vi "BattreyFGV.vi"(7 "Enum":enum16{"初始化", "讀取", "寫入", "閒置"}(ring), 10 "File Path":path=path "D:/battery/positive.txt", 11 "電池正負極陣列(輸入)":bool[](array[boolean])=[TRUE, TRUE, TRUE, TRUE, TRUE, TRUE, TRUE, TRUE, TRUE, TRUE, TRUE, TRUE, TRUE, TRUE, TRUE, TRUE, TRUE, TRUE, TRUE, TRUE, TRUE, TRUE, TRUE, TRUE, TRUE, TRUE, TRUE, TRUE, TRUE, TRUE, TRUE, TRUE, TRUE, TRUE, TRUE, TRUE, TRUE, TRUE, TRUE, TRUE]) -> (3 "電池正負極陣列(輸出)":bool[](array[boolean])=[TRUE, FALSE, TRUE, FALSE, TRUE, FALSE, TRUE, FALSE, TRUE, FALSE, TRUE, TRUE, FALSE, TRUE, FALSE, TRUE, FALSE, FALSE, TRUE, FALSE, TRUE, FALSE, TRUE, TRUE, FALSE, TRUE, FALSE, TRUE, FALSE, FALSE, TRUE, FALSE, TRUE, FALSE, TRUE, FALSE, TRUE, FALSE, TRUE, FALSE])   [LabVIEW 2015]
panel:
  in  "error In":errorcluster
  out "error out":errorcluster
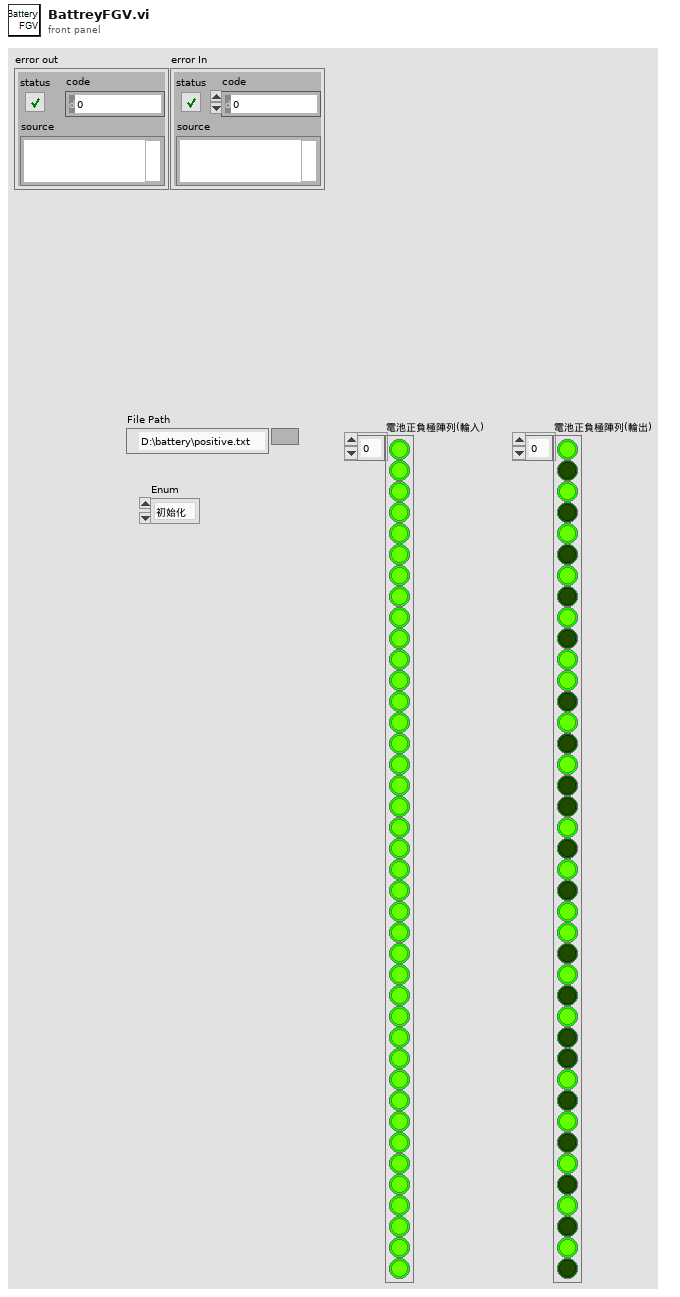
[diagram p1: front panel]
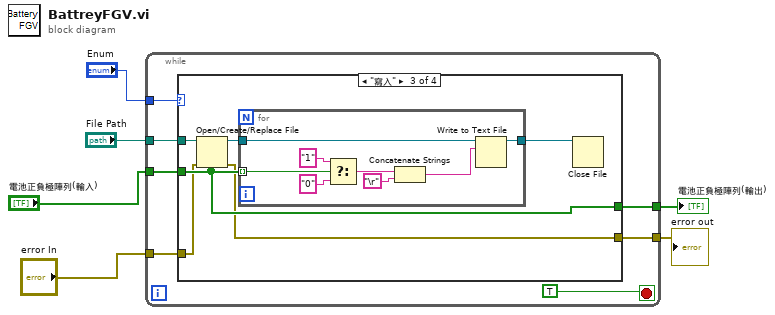
[diagram p0: block diagram]
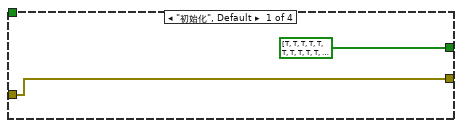
[diagram p2: hidden frame]
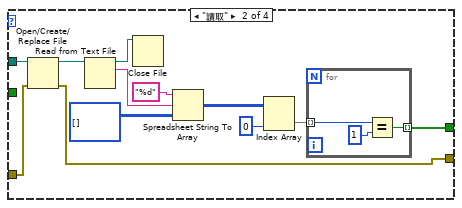
[diagram p3: hidden frame]
diagram:
  n1 = while {
    tunnel: "Enum" -> [w13]
    tunnel: "File Path" -> [w12]
    tunnel: [w11] -> w4
    tunnel: "電池正負極陣列(輸入)" -> [w10]
    tunnel: [w8] -> w2
    tunnel: "error In" -> [w7]
    stop <- TRUE stop-if-true
    n2 = case shown="\"寫入\"" w13 {
      tunnel: w12 -> [_ w19 w34 _]
      tunnel: [bool[] [TRUE, TRUE, TRUE, TRUE, TRUE, TRUE, TRUE, TRUE, TRUE, TRUE, TRUE, TRUE, TRUE, TRUE, TRUE, TRUE, TRUE, TRUE, TRUE, TRUE, TRUE, TRUE, TRUE, TRUE, TRUE, TRUE, TRUE, TRUE, TRUE, TRUE, TRUE, TRUE, TRUE, TRUE, TRUE, TRUE, TRUE, TRUE, TRUE, TRUE] ("電池正負極陣列(輸入)") w18 w33 w46] -> w11
      tunnel: w10 -> [_ _ w33 w46]
      tunnel: [w14 w17 w31 w45] -> w8
      tunnel: w7 -> [w14 w16 w32 w45]
      frame "初始化", Default {
      }
      frame "讀取" {
        n3 = Open/Create/Replace File(file path (use dialog)=w19, error in=w16) -> (refnum out=w25:refnum<file>, error out=w17:errorcluster)  [unwired: 4 in, 1 out]
        n4 = Read from Text File(file (use dialog)=w25) -> (refnum out=w22:refnum<file>, text=w27:string)  [unwired: 3 in, 2 out]
        n5 = Close File(refnum=w22) -> ()  [unwired: 1 in, 2 out]
        n6 = Spreadsheet String To Array(format string="%d", spreadsheet string=w27, array type (2D Dbl)=i32[][] []) -> (array=w21:i32[][])  [unwired: 1 in]
        n7 = Index Array(array=w21, index (col)=0 ("index (row)")) -> (element=w20:i32[])  [unwired: 1 in]
        n8 = for {
          tunnel: w20 -> [w30] mode=indexing
          tunnel: [w28] -> w18 mode=indexing
          n9 = Equal?(x=w30, y=1) -> (x = y?=w28:bool)
        }
      }
      frame "寫入" {
        n10 = Open/Create/Replace File(file path (use dialog)=w34, error in=w32) -> (refnum out=w36:refnum<file>, error out=w31:errorcluster)  [unwired: 4 in, 1 out]
        n11 = for {
          tunnel: w36 -> [w38]
          tunnel: w33 -> [w44] mode=indexing
          tunnel: [w37] -> w35
          n12 = Select(t="1", s=w44, f="0") -> (s? t:f=w41:string)
          n13 = Concatenate Strings(w41, "\r") -> (w39:string)
          n14 = Write to Text File(file (use dialog)=w38, text=w39) -> (refnum out=w37:refnum<file>)  [unwired: 2 in, 2 out]
        }
        n15 = Close File(refnum=w35) -> ()  [unwired: 1 in, 2 out]
      }
      frame "閒置" {
      }
    }
  }
  "電池正負極陣列(輸出)" <- w4
  "error out" <- w2
